vi "Eth Status Read Errors.vi"(7 "Status Reference":T1, 8 "error in (no error)":errorcluster, 10 "Lenght":i32, 11 "N":i32) -> (0 "error out":errorcluster, 1 "Errors":i32[](array[numeric]))   [LabVIEW 2021, in "Eth Status.lvlib"]
uses:
  Eth Status.lvlib
  Ctl/Status.ctl
  MB_TCP2/MB_TCP_State.ctl
  MB_TCP2/MB_TCP.lvclass
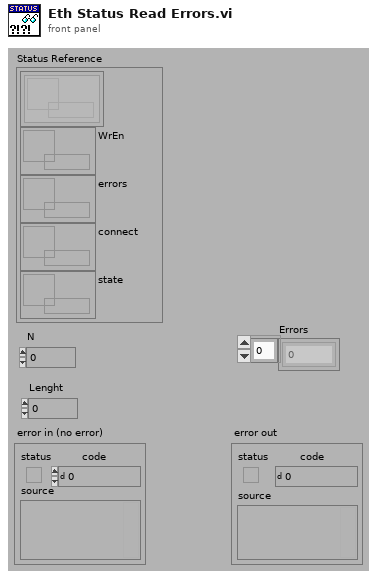
[diagram p1: front panel]
types:
  T1 = typedef "Eth Status.lvlib/Status.ctl" = cluster{"Set_states":refnum<queue>[], "WrEn":refnum<data-value>, "errors":refnum<data-value>, "connect":refnum<data-value>, "state":refnum<data-value>}
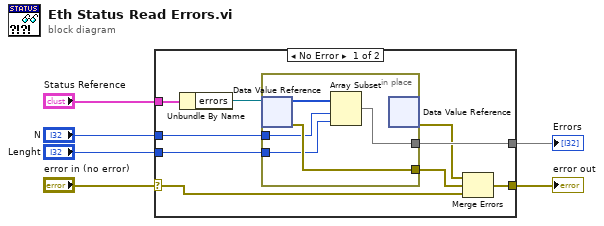
[diagram p0: block diagram]
diagram:
  n1 = case shown="No Error" "error in (no error)" {
    selector: "error in (no error)" -> [w7 w21]
    tunnel: [w12 w21] -> w6
    tunnel: [w15 _] -> w3
    tunnel: "N" -> [w14 _]
    tunnel: "Status Reference" -> [w13 _]
    tunnel: "Lenght" -> [w9 _]
    frame No Error {
      n2 = Unbundle By Name(w13) -> ("errors"=w8:refnum<data-value>)
      n3 = in-place {
        in-place-border: w14 -> [w18]
        in-place-border: [w16] -> w15
        in-place-border: [w20] -> w10
        in-place-border: w9 -> [w17]
        n4 = in-place-dvr #1(w8) -> (w19:i32[], w20:errorcluster)
        n5 = Array Subset(array=w19, index=w18, length=w17) -> (w16:i32[])
        n6 = in-place-dvr #1() -> (w11:errorcluster)  [unwired: 1 in, 1 out]
      }
      n7 = Merge Errors(w11, w10, w7) -> (w12:errorcluster)
    }
    frame Error {
    }
  }
  "error out" <- w6
  "Errors" <- w3
